vi "平行样集成干预数据组合(子VI).vi"(9 "污染物编码":string, 10 "数据输入":string[][](array[string]), 11 "小时数据发送次数":i32) -> (3 "输出组合":string)   [LabVIEW 2016, in "数据传输系统-05.lvlib"]
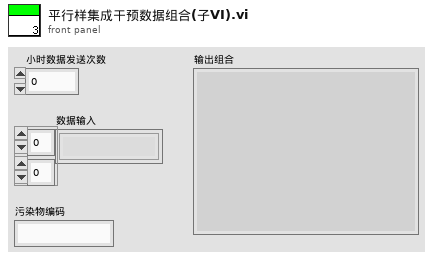
[diagram p1: front panel]
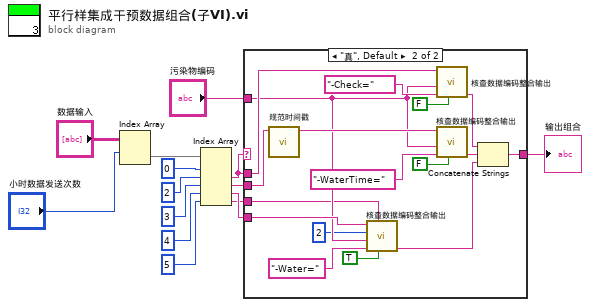
[diagram p0: block diagram]
diagram:
  n1 = Index Array(array="数据输入", index (row)="小时数据发送次数") -> (element=w7:string[])  [unwired: 1 in]
  n2 = Index Array(array=w7, index #1=0 ("索引"), index #2=2 ("索引"), index #3=3 ("索引"), index #4=4 ("索引"), index #5=5 ("索引")) -> (element #2=w4:string, element #3=w6:string, element #4=w5:string, element #5=w1:string)  [unwired: 1 out]
  n3 = case shown="\"真\", Default" w4 {
    selector: w4 -> [w15 _]
    tunnel: w4 -> [_ w32]
    tunnel: w5 -> [_ w26]
    tunnel: w6 -> [_ w24]
    tunnel: [w15 w19] -> w11
    tunnel: "污染物编码" -> [_ w18]
    tunnel: w1 -> [_ w16]
    frame "" {
    }
    frame "真", Default {
      n4 = call "规范时间戳.vi"("字符串"=w24) -> ("result string"=w23:string)  [unwired: 10 in]
      n5 = call "核查数据编码整合输出.vi"("字段结束"=TRUE, "数据标识"=w16, "数据类型"="-Water=", "污染物编码"=w18, "数据精度"=2, "数据值"=w26) -> ("编码输出"=w20:string)  [unwired: 5 in]
      n6 = call "核查数据编码整合输出.vi"("字段结束"=FALSE, "数据类型"="-Check=", "污染物编码"=w18, "数据值"=w32) -> ("编码输出"=w22:string)  [unwired: 7 in]
      n7 = call "核查数据编码整合输出.vi"("字段结束"=FALSE, "数据类型"="-WaterTime=", "污染物编码"=w18, "数据值"=w23) -> ("编码输出"=w21:string)  [unwired: 7 in]
      n8 = Concatenate Strings(w22, w21, w20) -> (w19:string)
    }
  }
  "输出组合" <- w11
